vi "Init.vi"(8 "error in (no error)":errorcluster, 10 "Init Data":variant, 11 "CryoCoolerAVC in":refnum<class "CryoCoolerAVC.lvclass">) -> (0 "error out":errorcluster, 2 "Channel List":refnum<class "HK Item.lvclass">[](array[class]), 3 "CryoCoolerAVC out":refnum<class "CryoCoolerAVC.lvclass">)   [LabVIEW 2024, in "CryoCoolerAVC.lvclass"]
uses:
  CryoCoolerAVC.lvclass
  hk-channel-class/hk-channel-class/HK Item/HK Item.lvclass
  CryoCoolerAVC.lvclass/CryoCoolerAVC.ctl
  Cryo Cooler.lvclass
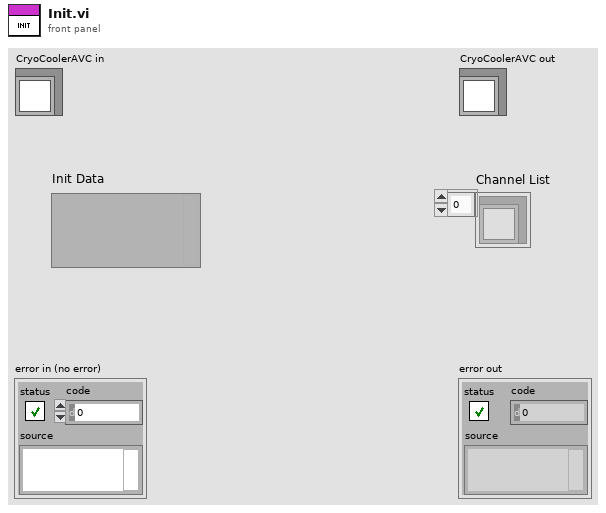
[diagram p1: front panel]
types:
  T1 = typedef "CryoCoolerAVC.lvclass/CryoCoolerAVC Settings.ctl" = cluster{"CryoTek 1 Addr":refnum<visa-resource-name>, "CryoTek 2 Addr":refnum<visa-resource-name>}
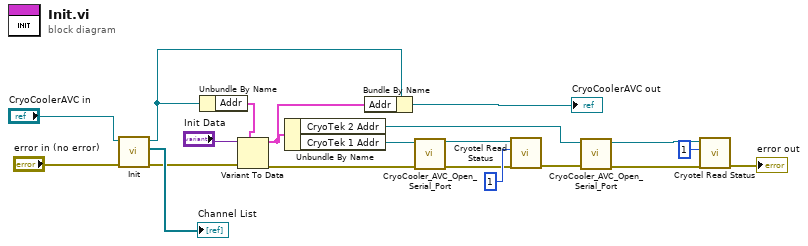
[diagram p0: block diagram]
diagram:
  n1 = call-parent "Init.vi"("error in (no error)"="error in (no error)", "Cryo Cooler in"="CryoCoolerAVC in") -> ("error out"=w17:errorcluster, "Channel List"=→"Channel List":refnum<class "HK Item.lvclass">[], "Cryo Cooler out"=w14:refnum<class "CryoCoolerAVC.lvclass">)  [unwired: 7 in]
  n2 = Unbundle By Name(w14) -> ("Addr"=w13:T1)
  n3 = Variant To Data(error in=w17, type=w13, Variant="Init Data") -> (data=w11:T1, error out=w7:errorcluster)
  n4 = Unbundle By Name(w11) -> ("CryoTek 2 Addr"=w3:refnum<visa-resource-name>, "CryoTek 1 Addr"=w8:refnum<visa-resource-name>)
  n5 = Bundle By Name(cluster=w14, "Addr"=w11) -> (→"CryoCoolerAVC out":refnum<class "CryoCoolerAVC.lvclass">)
  n6 = call "CryoCooler_AVC_Open_Serial_Port.vi"("error in (no error)"=w7, "VISA Resource (write)"=w8) -> ("error out"=w6:errorcluster, "VISA Resource out"=w4:refnum<visa-resource-name>)  [unwired: 8 in]
  n7 = call "Cryotel Read Status.vi"("error in"=w6, "Number of reads"=1, "VISA Resource (write)"=w4) -> ("error out"=w5:errorcluster)  [unwired: 6 in, 2 out]
  n8 = call "CryoCooler_AVC_Open_Serial_Port.vi"("error in (no error)"=w5, "VISA Resource (write)"=w3) -> ("error out"=w1:errorcluster, "VISA Resource out"=w2:refnum<visa-resource-name>)  [unwired: 8 in]
  n9 = call "Cryotel Read Status.vi"("error in"=w1, "Number of reads"=1, "VISA Resource (write)"=w2) -> ("error out"=→"error out":errorcluster)  [unwired: 6 in, 2 out]
